vi "LINAKReRead.vi"(8 "error in (no error)":errorcluster, 10 "LinakAddresses":u8[](array[numeric])) -> (0 "error out":errorcluster, 2 "AbsPositions":dbl[](array[numeric]), 3 "ThereYets":bool[](array[boolean]))   [LabVIEW 2021]
uses:
  LINAKUTIL.ctl
panel:
  out "Numeric":i32
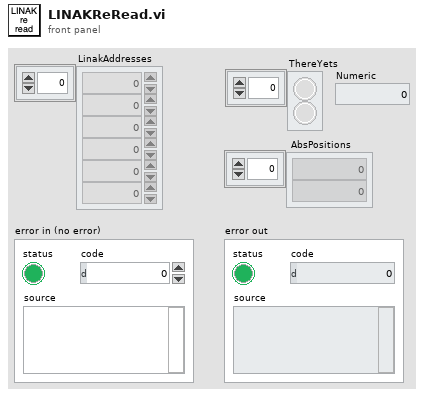
[diagram p1: front panel]
types:
  T1 = typedef "LINAKUTIL.ctl" = enum16{"Read", "ReadTarget", "WriteTarget", "SingleGo", "GlobalGo", "SafetySet", "WriteReadGo", "STOP"}
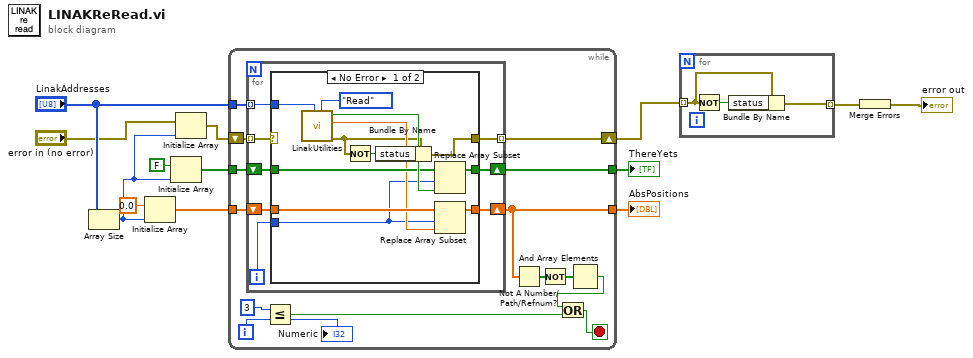
[diagram p0: block diagram]
diagram:
  n1 = Array Size(array="LinakAddresses") -> (size(s)=w6:i32)
  n2 = Initialize Array(0.0 ("element"), w6) -> (w8:dbl[])
  n3 = Initialize Array(FALSE, w6) -> (w7:bool[])
  n4 = Initialize Array("error in (no error)", w6) -> (w4:errorcluster[])
  n5 = while {
    tunnel: w8 -> [w27]
    tunnel: "LinakAddresses" -> [w26]
    tunnel: w7 -> [w25]
    tunnel: [w17] -> w13
    tunnel: [w16] -> w12
    shift-right: [w14] -> w3
    shift-left: w4 -> [w15]
    i -> [w24]
    stop <- w21 stop-if-true
    n6 = for {
      tunnel: w26 -> [w35] mode=indexing
      shift-right: [w33] -> w17
      shift-left: w27 -> [w34]
      shift-right: [w32] -> w16
      shift-left: w25 -> [w30]
      tunnel: w15 -> [w28] mode=indexing
      tunnel: [w29] -> w14 mode=indexing
      i -> [w31]
      n7 = case shown="No Error" w28 {
        selector: w28 -> [_ w48]
        tunnel: w35 -> [w46 _]
        tunnel: w34 -> [w45 w49]
        tunnel: [w44 w49] -> w33
        tunnel: [w43 w50] -> w32
        tunnel: w31 -> [w39 _]
        tunnel: w30 -> [w41 w50]
        tunnel: [w36 w48] -> w29
        frame No Error {
          n8 = call "LinakUtilities.vi"("LinakUtil"=LINAKUTIL."Read", "Linak Address"=w46) -> ("error out"=w37:errorcluster, "AbsPosition"=w40:dbl, "ThereYet?"=w42:bool)  [unwired: 6 in, 1 out]
          n9 = Not(x=w37) -> (.not. x?=w38:bool)
          n10 = Bundle By Name(cluster=w37, "status"=w38) -> (w36:errorcluster)
          n11 = Replace Array Subset(array=w41, new element=w42, index=w39) -> (w43:bool[])
          n12 = Replace Array Subset(array=w45, new element=w40, index=w39) -> (w44:dbl[])
        }
        frame Error {
        }
      }
    }
    n13 = Less Or Equal?(x=3, y=w24) -> (x <= y?=w19:bool)
    n14 = Not A Number/Path/Refnum?(number/path/refnum=w17) -> (NaN/Path/Refnum?=w22:bool[])
    n15 = Not(x=w22) -> (.not. x?=w20:bool[])
    n16 = And Array Elements(Boolean array=w20) -> (logical AND=w18:bool)
    n17 = Or(x=w18, y=w19) -> (x .or. y?=w21:bool)
    "Numeric" <- w24
  }
  "ThereYets" <- w12
  "AbsPositions" <- w13
  n18 = for {
    tunnel: w3 -> [w52] mode=indexing
    tunnel: [w51] -> w2 mode=indexing
    n19 = Not(x=w52) -> (.not. x?=w53:bool)
    n20 = Bundle By Name(cluster=w52, "status"=w53) -> (w51:errorcluster)
  }
  n21 = Merge Errors(w2) -> (→"error out":errorcluster)
